vi "niDDC temp - read FPGA debug info.vi"(8 "error in (no error)":errorcluster, 11 "Class in":refnum<class "7976R_v1.lvclass">) -> (0 "error out":errorcluster, 1 "FPGA FIFO overflow":bool, 2 "dma.overflow":bool, 3 "Class out":refnum<class "7976R_v1.lvclass">)   [LabVIEW 2015, in "7976R_v1.lvclass"]
uses:
  <userlib>/SE-APP-Receiver/NI5772/7976R_v1/7976R_v1.lvclass
  <userlib>/SE-APP-Receiver/NI5772/7976R_v1/7976R_v1.lvclass/7976R_v1.ctl
  <vilib>/Utility/error.llb/Error Cluster From Error Code.vi
  <vilib>/rvi/errors/niLvFpgaAdjustHostInterfaceError.vi
  <vilib>/rvi/interface/nirviReadWriteControl/nirviReadWriteControl.xnode
  <userlib>/SE-APP-Receiver/NI5772/7976R_v1/Private/FPGA VI Reference_DDC_v1.8.ctl
  NiFpgaLv.dll
  <vilib>/rvi/interface/Simulation/niFpgaSimulationCallBeginRW.vi
panel:
  out "Halfband dec":dbl=0.9999993983124225
  out "(cntr1/cntr5)/dec_factor":dbl=1.585684148108468e-07
  out "cntr1/cntr2":dbl=2.0000007517953082
  out "dbg.cntr.rdy_f_in":u64=1
  out "dbg.cntr.2b":u64=821028916
  out "dbg.cntr.1b":u64=4166034927
  out "dbg.2":T1={"I"=7.62939453125e-06, "Q"=0.00196075439453125, "overflow"=FALSE} {"I" format="%.18g"; "Q" format="%.18g"}
  out "dbg.1":T2(array[cluster])=[{"I"=0.05419921875, "Q"=0.05419921875, "overflow"=FALSE}, {"I"=0.0576171875, "Q"=0.0576171875, "overflow"=FALSE}, {"I"=0.05859375, "Q"=0.05859375, "overflow"=FALSE}, {"I"=0.01904296875, "Q"=0.01904296875, "overflow"=FALSE}, {"I"=-0.05908203125, "Q"=-0.05908203125, "overflow"=FALSE}, {"I"=-0.06201171875, "Q"=-0.06201171875, "overflow"=FALSE}, {"I"=-0.0595703125, "Q"=-0.0595703125, "overflow"=FALSE}, {"I"=-0.02294921875, "Q"=-0.02294921875, "overflow"=FALSE}] {"I" format="%.18g"; "Q" format="%.18g"}
  out "dbg.cntr.1":u64=4166029160
  out "dbg.cntr.2":u64=2083013797
  out "dbg.cntr.3":u64=821024097
  out "dbg.cntr.4":u64=821023603
  out "dbg.cntr.5":u64=8210228
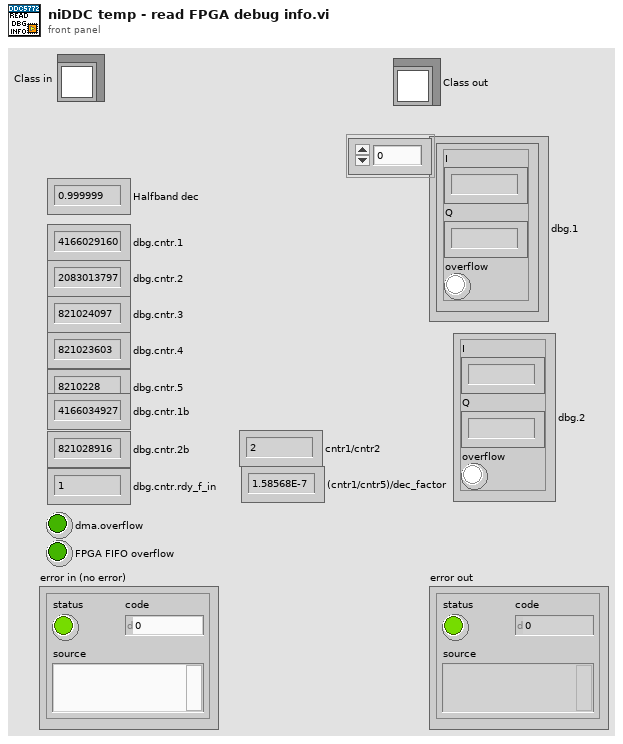
[diagram p1: front panel]
types:
  T1 = cluster{"I":fxp<+/-,18,1>, "Q":fxp<+/-,18,1>, "overflow":bool}
  T2 = cluster{"I":fxp<+/-,18,1>, "Q":fxp<+/-,18,1>, "overflow":bool}[]
  T3 = typedef "7976R_v1.lvclass/FPGA VI Reference_DDC_v1.8.ctl" = refnum<k20>
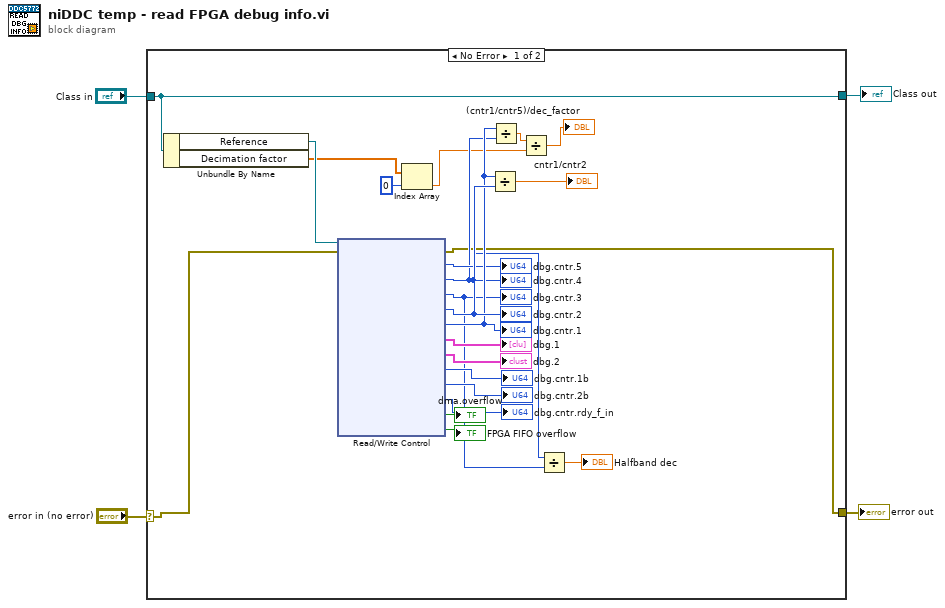
[diagram p0: block diagram]
diagram:
  n1 = case shown="No Error" "error in (no error)" {
    selector: "error in (no error)" -> [w9 w29]
    tunnel: [w8 w29] -> w4
    tunnel: "Class in" -> [w11 w28]
    tunnel: [w11 w28] -> w1
    frame No Error {
      n2 = Unbundle By Name(w11) -> ("Reference"=w10:T3, "Decimation factor"=w7:dbl[])
      n3 = xnode "Read/Write Control"("FPGA VI Reference In"=w10, "error in"=w9) -> ("error out"=w8:errorcluster, "dbg.cntr.5"=→"dbg.cntr.5":u64, "dbg.cntr.4"=w16:u64, "dbg.cntr.3"=w15:u64, "dbg.cntr.2"=w22:u64, "dbg.cntr.1"=w20:u64, "dbg.1"=→"dbg.1":T2, "dbg.2"=→"dbg.2":T1, "dbg.cntr.1b"=→"dbg.cntr.1b":u64, "dbg.cntr.2b"=→"dbg.cntr.2b":u64, "dbg.cntr.rdy_f_in"=→"dbg.cntr.rdy_f_in":u64, "dma.overflow"=→"dma.overflow":bool, "fifo.0.of"=→"FPGA FIFO overflow":bool)  [unwired: 1 out]
      "dbg.cntr.4" <- w16
      "dbg.cntr.3" <- w15
      "dbg.cntr.2" <- w22
      "dbg.cntr.1" <- w20
      n4 = Index Array(array=w7, index=0) -> (element=w6:dbl)
      n5 = Divide(x=w20, y=w22) -> (x/y=→"cntr1/cntr2":dbl)
      n6 = Divide(x=w20, y=w16) -> (x/y=w18:dbl)
      n7 = Divide(x=w18, y=w6) -> (x/y=→"(cntr1/cntr5)/dec_factor":dbl)
      n8 = Divide(x=w16, y=w15) -> (x/y=→"Halfband dec":dbl)
    }
    frame Error {
    }
  }
  "error out" <- w4
  "Class out" <- w1
